vi "Register.vi"(11 "Event in":refnum<class "Event.lvclass">) -> (2 "Registration":refnum<event-registration>, 3 "Event out":refnum<class "Event.lvclass">)   [LabVIEW 2021, in "jettl.lvlib" / "Event.lvclass"]
uses:
  Event.lvclass
  Msg Strategy/Msg Strategy.lvclass
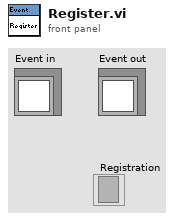
[diagram p1: front panel]
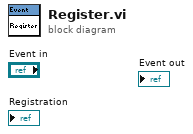
[diagram p0: block diagram]
diagram:
